vi "CustomError.vi"(7 "Error Selector":T1, 8 "error in (no error)":errorcluster, 10 "VI name":string) -> (0 "error out":errorcluster)   [LabVIEW 2017, in "WaveformTask.lvclass"]
uses:
  WaveformTask.lvclass
  ErrorSelector.ctl
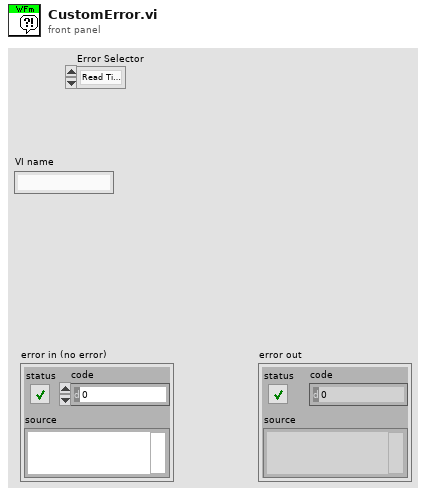
[diagram p1: front panel]
types:
  T1 = typedef "WaveformTask.lvclass/ErrorSelector.ctl" = enum16{"Read Timeout", "Module Underflow", "DMA Overflow", "Chan Count", "Run Timeout", "Start Timeout", "Stop Timeout"}
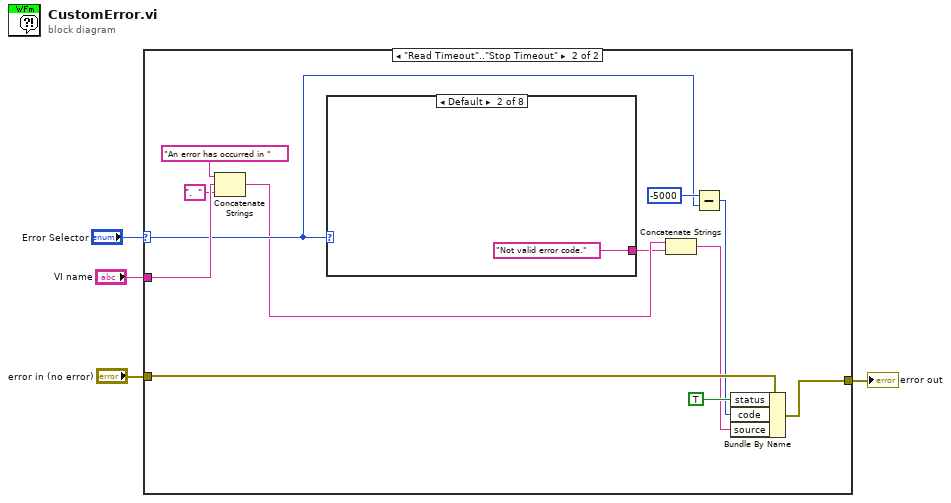
[diagram p0: block diagram]
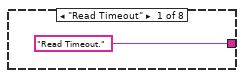
[diagram p3: hidden frame]
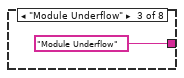
[diagram p4: hidden frame]
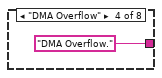
[diagram p5: hidden frame]
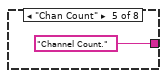
[diagram p6: hidden frame]
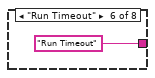
[diagram p7: hidden frame]
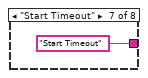
[diagram p8: hidden frame]
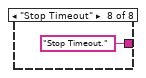
[diagram p9: hidden frame]
diagram:
  n1 = case shown="\"Read Timeout\"..\"Stop Timeout\"" "Error Selector" {
    selector: "Error Selector" -> [_ w11]
    tunnel: "error in (no error)" -> [w5 w14]
    tunnel: [w5 w9] -> w3
    tunnel: "VI name" -> [_ w16]
    frame Default {
    }
    frame "Read Timeout".."Stop Timeout" {
      n2 = Concatenate Strings("An error has occurred in " ("string"), w16, ".  " ("string")) -> (w8:string)
      n3 = case shown="Default" w11 {
        tunnel: ["Read Timeout." "Not valid error code." "Module Underflow" "DMA Overflow." "Channel Count." "Run Timeout" "Start Timeout" "Stop Timeout."] -> w7
        frame "Read Timeout" {
        }
        frame Default {
        }
        frame "Module Underflow" {
        }
        frame "DMA Overflow" {
        }
        frame "Chan Count" {
        }
        frame "Run Timeout" {
        }
        frame "Start Timeout" {
        }
        frame "Stop Timeout" {
        }
      }
      n4 = Concatenate Strings(w8, w7) -> (w6:string)
      n5 = Subtract(x=-5000, y=w11) -> (x-y=w10:i32)
      n6 = Bundle By Name(cluster=w14, "status"=TRUE, "code"=w10, "source"=w6) -> (w9:errorcluster)
    }
  }
  "error out" <- w3
